vi "niFPGA Look-Up Table 1D.vi"(0 "address":u16, 3 "fractional index (x 2^16)":u16) -> (7 "data out":i16)   [LabVIEW 2017]
doc: "Provides a general-purpose block of initialized memory. Use look-up tables to store waveforms for signal generation, to model nonlinear systems, and for arithmetic computations. If you use the Look-Up Table 1D Express VI in a single-cycle Timed Loop, wire the outputs directly to Feedback Nodes. The Look-Up Table 1D Express VI takes an entire clock cycle to execute in a single-cycle Timed Loop."
panel:
  in  "Init data":i32[](array[numeric])
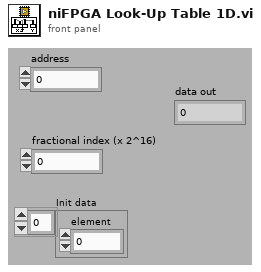
[diagram p1: front panel]
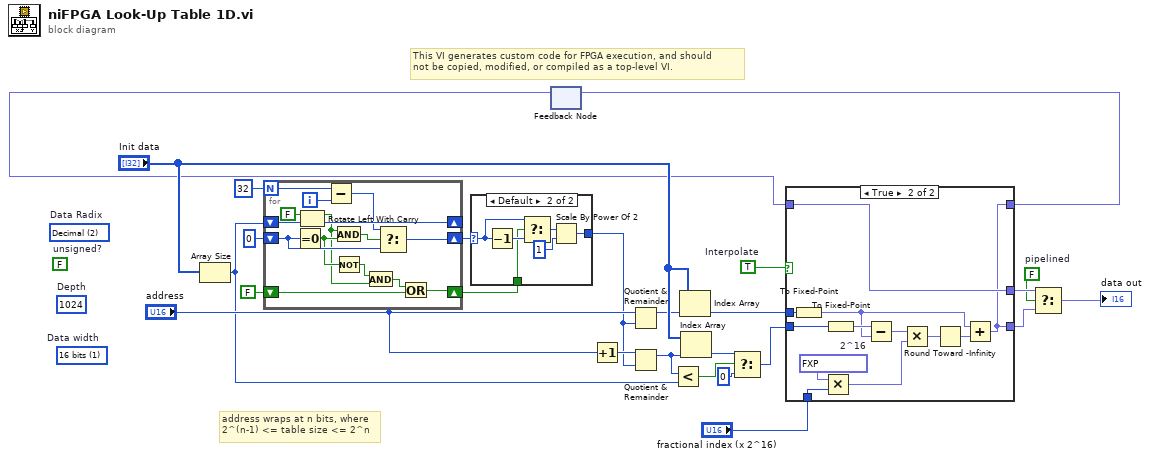
[diagram p0: block diagram]
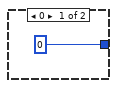
[diagram p2: hidden frame]
diagram:
  w11 = FALSE  # pipelined
  (unwired) 1024  # Depth
  (unwired) u8 1 items=["8 bits", "16 bits", "32 bits"]  # Data width
  (unwired) FALSE  # unsigned?
  (unwired) u8 2 items=["Binary", "Octal", "Decimal", "Hexadecimal"]  # Data Radix
  w22 = TRUE  # Interpolate
  # "address wraps at n bits, where\n2^(n-1) <= table size <= 2^n"
  # "This VI generates custom code for FPGA execution, and should\nnot be copied, modified, or compiled as a top-level VI."
  n1 = Array Size(array="Init data") -> (size(s)=w6:i32)
  n2 = for {
    N: 32 -> [w38]
    shift-right: [w32] -> w5
    shift-left: 0 ("size(s)") -> [w33]
    shift-right: [w36] -> _
    shift-left: w6 -> [w40]
    shift-right: [w26] -> w4
    shift-left: FALSE -> [w27]
    i -> [w37]
    n3 = Equal To 0?(x=w33) -> (x = 0?=w31:bool)
    n4 = Rotate Left With Carry(2:w40, 3:FALSE ("carry")) -> (0:w36:i32, 1:w29:bool)
    n5 = Subtract(x=w38, y=w37) -> (x-y=w34:i32)
    n6 = And(x=w29, y=w31) -> (x .and. y?=w35:bool)
    n7 = Not(x=w31) -> (.not. x?=w30:bool)
    n8 = And(x=w30, y=w29) -> (x .and. y?=w28:bool)
    n9 = Select(t=w34, s=w35, f=w33) -> (s? t:f=w32:i32)
    n10 = Or(x=w28, y=w27) -> (x .or. y?=w26:bool)
  }
  n11 = case shown="Default" w5 {
    selector: w5 -> [_ w43]
    tunnel: [0 w45] -> w3
    tunnel: w4 -> [_ w42]
    frame 0 {
    }
    frame Default {
      n12 = Decrement(x=w43) -> (x-1=w44:i32)
      n13 = Select(t=w43, s=w42, f=w44) -> (s? t:f=w47:i32)
      n14 = Scale By Power Of 2(n=w47, x=1 ("size(s)")) -> (x*2^n=w45:i32)
    }
  }
  n15 = feedback #1() -> (w1:fxp<+/-,48,48>)  [unwired: 1 in]
  n16 = Increment(x="address") -> (x+1=w23:u16)
  n17 = Quotient & Remainder(x="address", y=w3) -> (x-y*floor(x/y)=w19:i32)  [unwired: 1 out]
  n18 = Quotient & Remainder(x=w23, y=w3) -> (x-y*floor(x/y)=w18:i32)  [unwired: 1 out]
  n19 = Less?(x=w18, y=w6) -> (x < y?=w16:bool)
  n20 = Index Array(array="Init data", index=w19) -> (element=w24:i32)
  n21 = Index Array(array="Init data", index=w18) -> (element=w17:i32)
  n22 = Select(t=w17, s=w16, f=0) -> (s? t:f=w14:i32)
  n23 = case shown="True" w22 {
    tunnel: "fractional index (x 2^16)" -> [_ w52]
    tunnel: [w49 w53] -> w12
    tunnel: w24 -> [w49 w60]
    tunnel: w14 -> [_ w59]
    tunnel: [w49 w53] -> w2
    tunnel: w1 -> [w48 w61]
    tunnel: [w48 w61] -> w13
    frame False {
    }
    frame True {
      w50 = fxp<+/-,16,0> 1.52587890625e-05  # 2^16
      n24 = To Fixed-Point(number=w60) -> (fixed-point=w54:fxp<+/-,32,32>)  [unwired: 1 in]
      n25 = Multiply(x=w50, y=w52) -> (x*y=w51:fxp<+/-,32,16>)
      n26 = To Fixed-Point(number=w59) -> (fixed-point=w58:fxp<+/-,32,32>)  [unwired: 1 in]
      n27 = Subtract(x=w58, y=w54) -> (x-y=w57:fxp<+/-,33,33>)
      n28 = Multiply(x=w57, y=w51) -> (x*y=w56:fxp<+/-,64,48>)
      n29 = Round Toward -Infinity(1:w56) -> (0:w55:fxp<+/-,48,48>)
      n30 = Add(x=w54, y=w55) -> (x+y=w53:fxp<+/-,48,48>)
    }
  }
  n31 = feedback-in #1(w2) -> ()
  n32 = Select(t=w13, s=w11, f=w12) -> (s? t:f=→"data out":fxp<+/-,48,48>)
